vi "BME_DG_SetClock.vi"(5 "ClockEnable":bool, 7 "ClockSource":T1=1 items=["Internal Oscillator"=1, "External Trigger"=2, "Trigger-> Oscillator"=3, "MasterSlave Bus"=4], 8 "error in (no error)":errorcluster, 9 "External Trigger Modulo":u16=8, 10 "Internal Osci Modulo":u16=8, 11 "DG_NumberM":i32) -> (0 "error out":errorcluster)   [LabVIEW 2009, in "POLARIS BME DG.lvlib"]
uses:
  POLARIS BME DG.lvlib
  ClockSource.ctl
  BME DLL/DelayGenerator.dll
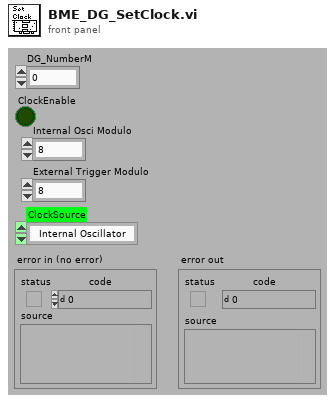
[diagram p1: front panel]
types:
  T1 = typedef "POLARIS BME DG.lvlib/ClockSource.ctl" = i32
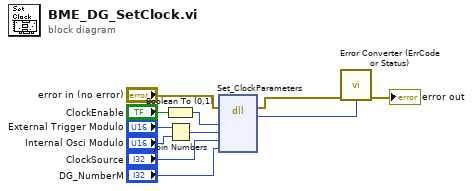
[diagram p0: block diagram]
diagram:
  n1 = Boolean To (0,1)(Boolean="ClockEnable") -> (0, 1=w8:i16)
  n2 = Join Numbers(hi="External Trigger Modulo", lo="Internal Osci Modulo") -> ((hi.lo)=w1:u32)
  n3 = dll-call lib="C:/CS Framework/LVSCC/LV2009/GPL/Projects/cs-framework/CSClass/CSPOLARIS/POLARIS BME DG/BME DLL/DelayGenerator.dll" fn="Set_ClockParameters"(error in="error in (no error)", "ClockEnable"=w8, "DivideBy"=w1, "ClockSource"="ClockSource", "DG_Number"="DG_NumberM") -> (error out=w6:errorcluster, w4:i32)  [unwired: 6 in, 1 out]
  n4 = call "Error Converter (ErrCode or Status).vi"("error in (no error)"=w6, "error code"=w4) -> ("error out"=→"error out":errorcluster)  [unwired: 9 in]
